vi "Values as Strings.vi"(8 "error in (no error)":errorcluster, 11 "GroupAbstract in":refnum<class "GroupAbstract.lvclass">) -> (0 "error out":errorcluster, 2 "Value Strings":string[](array[string]), 3 "GroupAbstract out":refnum<class "GroupAbstract.lvclass">)   [LabVIEW 2020, in "Vecto.lvlib" / "GroupAbstract.lvclass"]
uses:
  GroupAbstract.lvclass
  GroupAbstract.lvclass/GroupAbstract.ctl
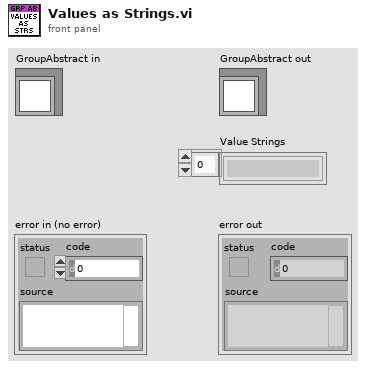
[diagram p1: front panel]
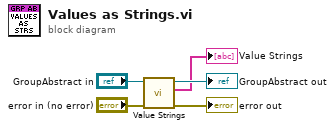
[diagram p0: block diagram]
diagram:
  n1 = call-dynamic "Value Strings.vi"("error in (no error)"="error in (no error)", "GroupAbstract in"="GroupAbstract in") -> ("error out"=→"error out":errorcluster, "Value Strings"=→"Value Strings":string[], "GroupAbstract out"=→"GroupAbstract out":refnum<class "GroupAbstract.lvclass">)  [unwired: 7 in]
